vi "build event cluster start.vi"() -> ()   [LabVIEW 2014]
uses:
  typedefs/event cluster typedef.ctl
  typedefs/time cluster typedef.ctl
panel:
  in  "time cluster in":T1
  in  "position in [km]":sgl
  out "event data out":T2
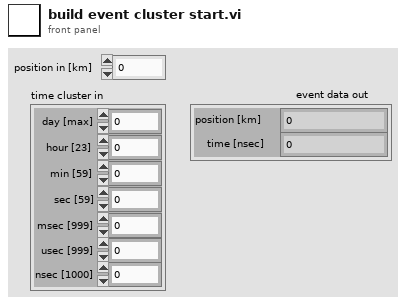
[diagram p1: front panel]
types:
  T1 = typedef "time cluster typedef.ctl" = cluster{"day [max]":u32, "hour [23]":u32, "min [59]":u32, "sec [59]":u32, "msec [999]":u32, "usec [999]":u32, "nsec [1000]":u32}
  T2 = typedef "event cluster typedef.ctl" = cluster{"position [km]":sgl, "time [nsec]":i64}
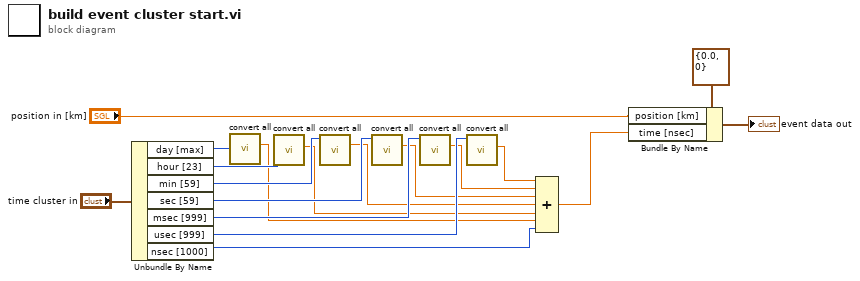
[diagram p0: block diagram]
diagram:
  n1 = Unbundle By Name("time cluster in") -> ("day [max]"=w14:u32, "hour [23]"=w13:u32, "min [59]"=w12:u32, "sec [59]"=w11:u32, "msec [999]"=w10:u32, "usec [999]"=w9:u32, "nsec [1000]"=w8:u32)
  n2 = call "convert all.vi"("Time"=w14) -> ("day to nsec"=w1:dbl)  [unwired: 10 in]
  n3 = call "convert all.vi"("Time"=w13) -> ("day to nsec"=w2:dbl)  [unwired: 10 in]
  n4 = call "convert all.vi"("Time"=w12) -> ("day to nsec"=w3:dbl)  [unwired: 10 in]
  n5 = call "convert all.vi"("Time"=w11) -> ("day to nsec"=w4:dbl)  [unwired: 10 in]
  n6 = call "convert all.vi"("Time"=w10) -> ("day to nsec"=w5:dbl)  [unwired: 10 in]
  n7 = call "convert all.vi"("Time"=w9) -> ("day to nsec"=w6:dbl)  [unwired: 10 in]
  n8 = Compound Arithmetic op=ADD(w6, w5, w4, w3, w2, w1, w8) -> (w7:dbl)
  n9 = Bundle By Name(cluster=T2 {"position [km]"=0.0, "time [nsec]"=0} ("event data out"), "position [km]"="position in [km]", "time [nsec]"=w7) -> (→"event data out":T2)
